vi "1d Average Filter.vi"(9 "Filter Width":i32, 11 "Unfiltered Data":dbl[](array[numeric])) -> (3 "Filtered data out":dbl[](array[numeric]))   [LabVIEW 2013]
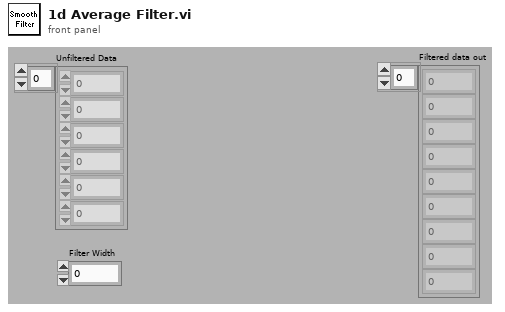
[diagram p1: front panel]
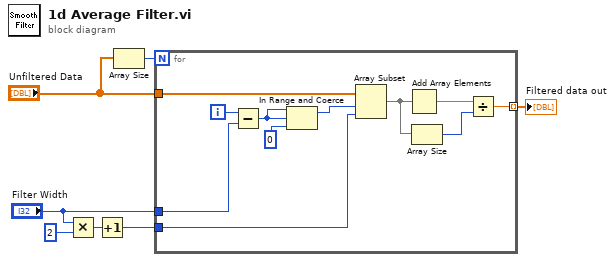
[diagram p0: block diagram]
diagram:
  n1 = Multiply(x="Filter Width", y=2) -> (x*y=w5:i32)
  n2 = Increment(x=w5) -> (x+1=w4:i32)
  n3 = Array Size(array="Unfiltered Data") -> (size(s)=w2:i32)
  n4 = for {
    N: w2 -> [_]
    tunnel: "Unfiltered Data" -> [w18]
    tunnel: "Filter Width" -> [w16]
    tunnel: w4 -> [w12]
    tunnel: [w8] -> w3 mode=indexing
    i -> [w17]
    n5 = Subtract(x=w17, y=w16) -> (x-y=w15:i32)
    n6 = In Range and Coerce(upper limit=w15, x=w15, lower limit=0) -> (coerced(x)=w13:i32)  [unwired: 1 out]
    n7 = Array Subset(array=w18, index=w13, length=w12) -> (w10:dbl[])
    n8 = Add Array Elements(numeric array=w10) -> (sum=w11:dbl)
    n9 = Array Size(array=w10) -> (size(s)=w9:i32)
    n10 = Divide(x=w11, y=w9) -> (x/y=w8:dbl)
  }
  "Filtered data out" <- w3
